vi "运维调试.vi"() -> ()   [LabVIEW 2016]
uses:
  <vilib>/Utility/miscctls.llb/LVPointTypeDef.ctl
  PLC/PLC.lvlib
panel:
  in  "运维调试单选按钮":T1(xcontrol)
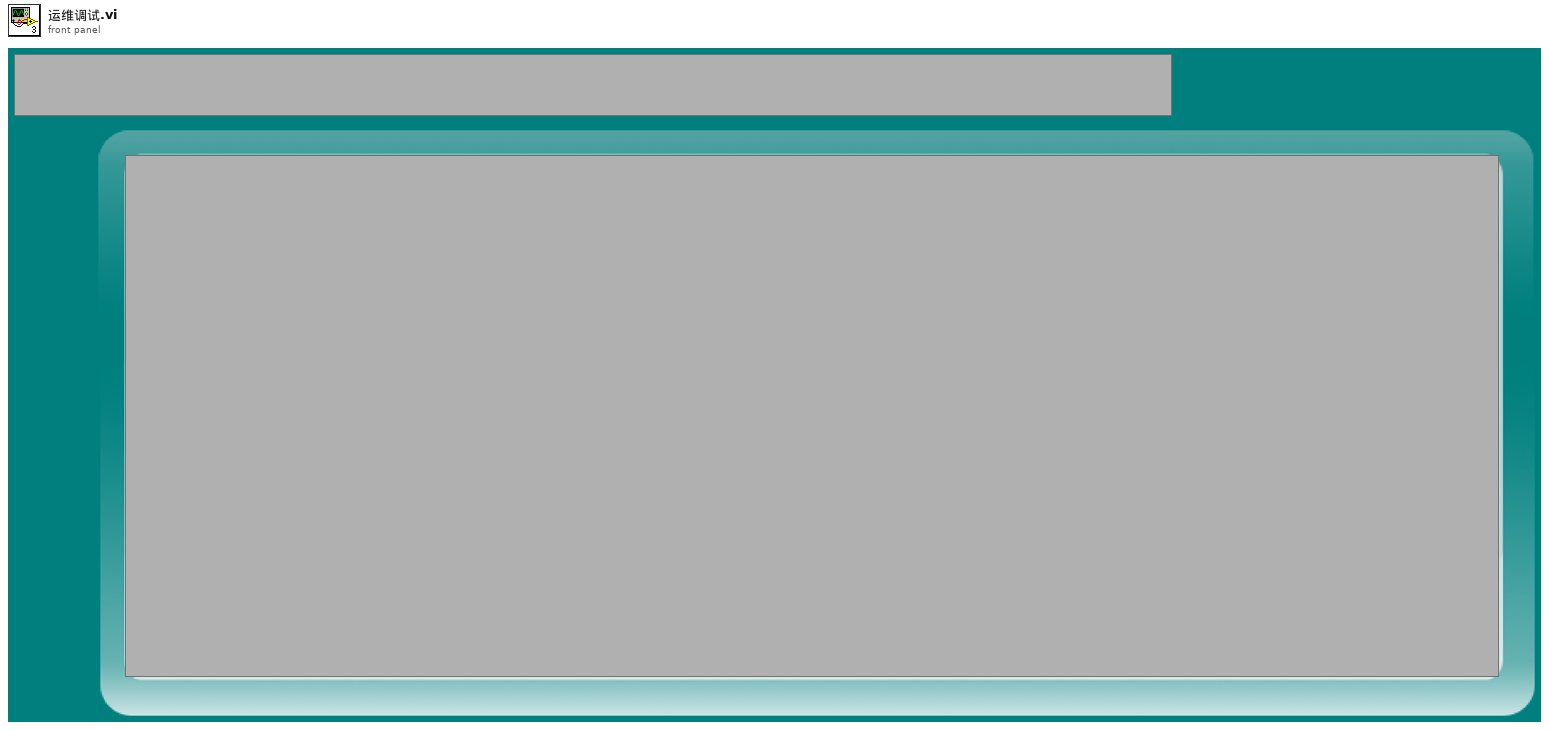
[diagram p1: front panel]
types:
  T1 = enum16{"采配水", "CODmn", "氨氮", "总磷总氮", "多参数", "质控单元", "其他"}
  T2 = typedef "LVPointTypeDef.ctl" = cluster{"Horizontal":i16, "Vertical":i16}
  T3 = enum32{"Bad", "Idle", "Run top level", "Running"}
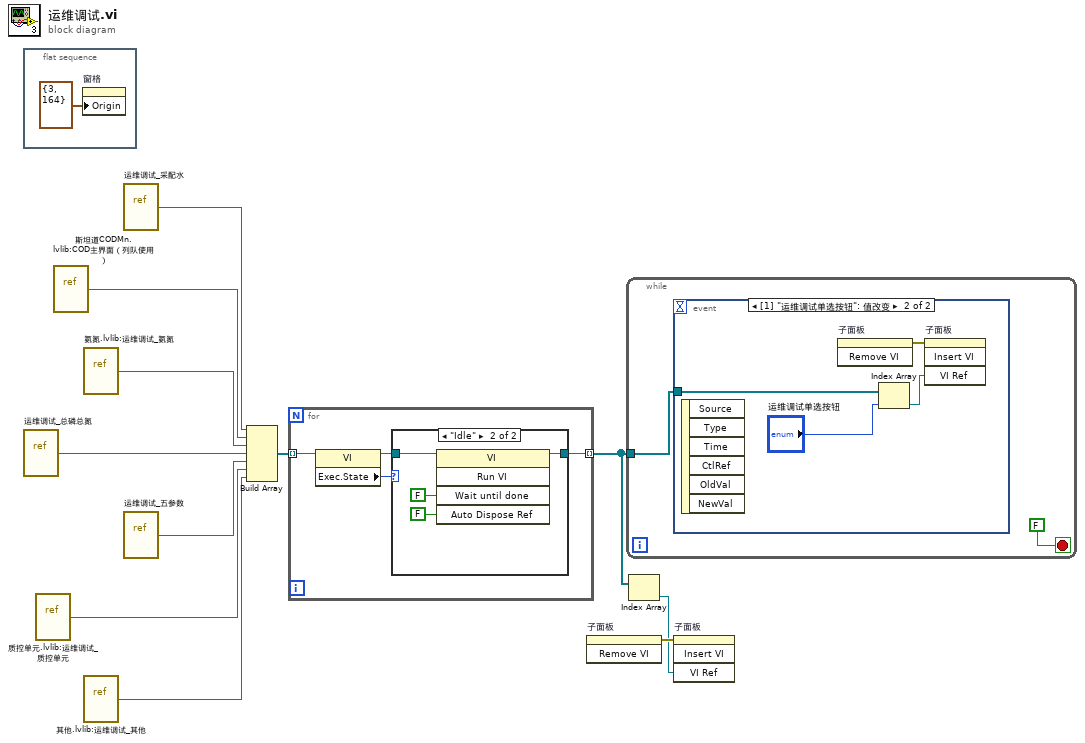
[diagram p0: block diagram]
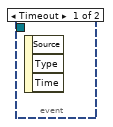
[diagram p3: hidden frame]
diagram:
  n1 = flat-sequence {
    frame #0 {
      n2 = property on="窗格" class="Pane"("Origin"=T2 {"Horizontal"=3, "Vertical"=164} ("原点")) -> ()  [unwired: 2 in, 2 out]
    }
  }
  n3 = vi-ref "运维调试_总磷总氮.vi"() -> (w4:refnum<vi>)
  n4 = vi-ref "质控单元.lvlib:运维调试_质控单元.vi"() -> (w2:refnum<vi>)
  n5 = vi-ref "斯坦道CODMn.lvlib:COD主界面（列队使用）.vi"() -> (w5:refnum<vi>)
  n6 = vi-ref "氨氮.lvlib:运维调试_氨氮.vi"() -> (w1:refnum<vi>)
  n7 = vi-ref "其他.lvlib:运维调试_其他.vi"() -> (w3:refnum<vi>)
  n8 = vi-ref "运维调试_采配水.vi"() -> (w8:refnum<vi>)
  n9 = vi-ref "运维调试_五参数.vi"() -> (w7:refnum<vi>)
  n10 = Build Array(w8, w5, w1, w4, w7, w2, w3) -> (w6:refnum<vi>[])
  n11 = for {
    tunnel: w6 -> [w16] mode=indexing
    tunnel: [w13] -> w10 mode=indexing
    n12 = property class="VI"(reference=w16) -> (reference out=w14:refnum<vi>, "Exec.State"=w15:T3)  [unwired: 1 in, 1 out]
    n13 = case shown="\"Idle\"" w15 {
      tunnel: w14 -> [w17 w19]
      tunnel: [w17 w18] -> w13
      frame "Bad", Default {
      }
      frame "Idle" {
        n14 = invoke class="VI" method="Run VI"(reference=w19, "Wait until done"=FALSE ("结束前等待"), "Auto Dispose Ref"=FALSE ("自动销毁引用")) -> (reference out=w18:refnum<vi>)  [unwired: 2 in, 4 out]
      }
    }
  }
  n15 = invoke on="子面板" class="SubPnl" method="Remove VI"() -> (error out=w11:errorcluster)  [unwired: 3 in, 2 out]
  n16 = while {
    tunnel: w10 -> [w22]
    stop <- FALSE stop-if-true
    n17 = event shown="[1] \"运维调试单选按钮\": 值改变" {
      selector: _ -> [_ _]
      dyn-events: _ -> [_ _]
      timeout: _ -> [_ _]
      tunnel: w22 -> [_ w25]
      event Timeout {
        n18 = event-data() -> ()  [unwired: 1 in, 3 out]
      }
      event "运维调试单选按钮": Value Change {
        n19 = event-data() -> ()  [unwired: 1 in, 6 out]
        n20 = invoke on="子面板" class="SubPnl" method="Remove VI"() -> (error out=w27:errorcluster)  [unwired: 3 in, 2 out]
        n21 = Index Array(array=w25, index="运维调试单选按钮") -> (element=w24:refnum<vi>)
        n22 = invoke on="子面板" class="SubPnl" method="Insert VI"(error in=w27, "VI Ref"=w24) -> ()  [unwired: 2 in, 4 out]
      }
    }
  }
  n23 = Index Array(array=w10) -> (element=w9:refnum<vi>)  [unwired: 1 in]
  n24 = invoke on="子面板" class="SubPnl" method="Insert VI"(error in=w11, "VI Ref"=w9) -> ()  [unwired: 2 in, 4 out]
